vi "_WriteAttributes.vi"(2 "attribute Values":T1(array[cluster]), 3 "device name":string) -> (0 "error stack":string[](array[string]), 1 "error code":i32)   [LabVIEW 2014, in "tango.lvlib"]
uses:
  tango.lvlib
  tango_binding.so
panel:
  # "This Vi is deprecated and only maintained for backward compatibility. Please use  _TangoWriteAttributes instead."
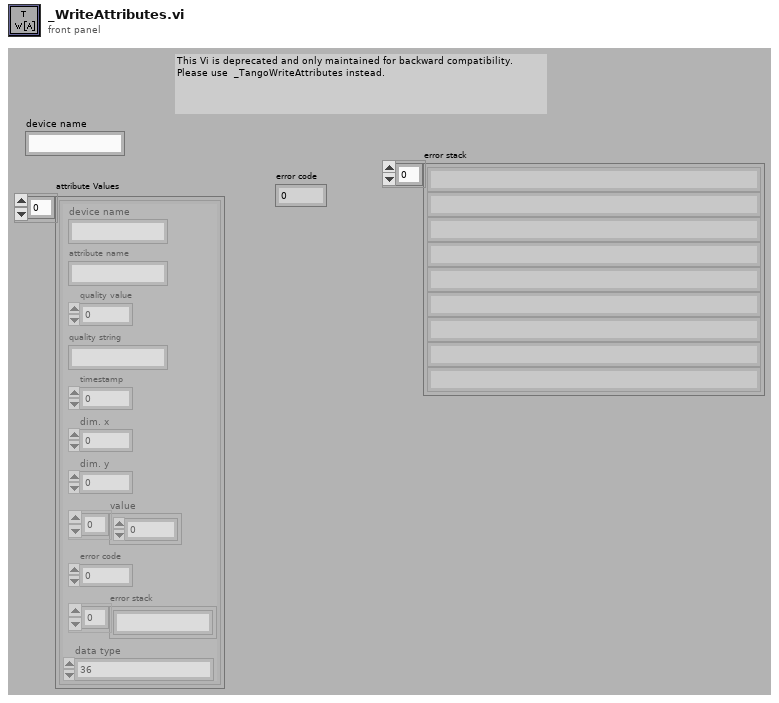
[diagram p1: front panel]
types:
  T1 = cluster{"device name":string, "attribute name":string, "quality value":i16, "quality string":string, "timestamp":dbl, "dim. x":i32, "dim. y":i32, "value":u8[], "error code":i32, "error stack":string[], "data type":u16}[]
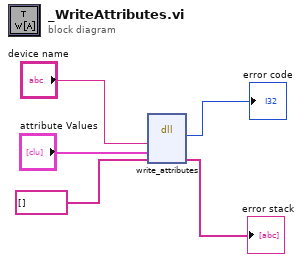
[diagram p0: block diagram]
diagram:
  n1 = dll-call lib="tango_binding.*" fn="write_attributes"("device_name"="device name", "attr_values_inout"="attribute Values", "error_stack"=string[] [] ("error stack")) -> ("type de retour"=→"error code":i32, "error_stack"=→"error stack":string[])  [unwired: 5 in, 2 out]
